vi "Get Project Info.vi"(8 "error in (no error)":errorcluster, 11 "Project Inspector in":refnum<class "Project Inspector.lvclass">) -> (0 "error out":errorcluster, 1 "Path":path, 2 "Name":string, 3 "Project Inspector out":refnum<class "Project Inspector.lvclass">, 4 "Item Paths":path[](array[path]))   [LabVIEW 2017, in "Cobertura.lvlib" / "Project Inspector.lvclass"]
uses:
  Project Inspector.lvclass
  Project Inspector.lvclass/Project Inspector.ctl
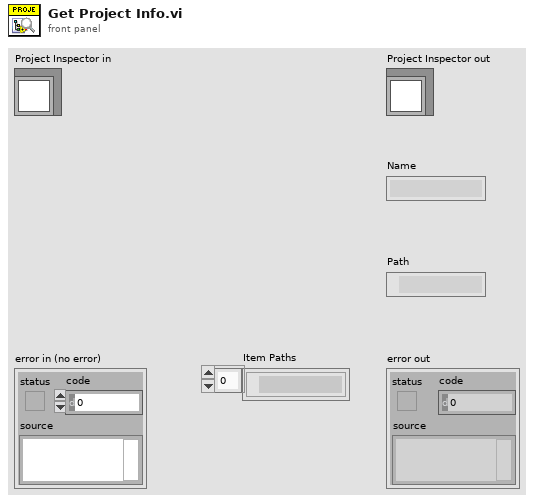
[diagram p1: front panel]
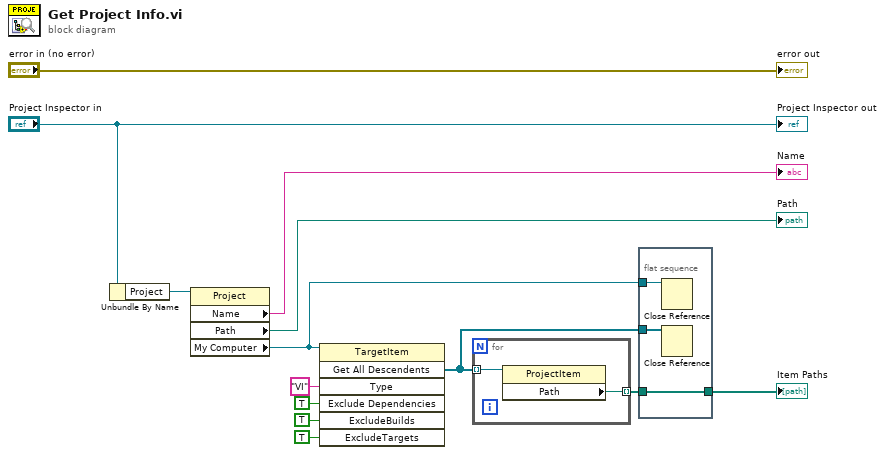
[diagram p0: block diagram]
diagram:
  n1 = Unbundle By Name("Project Inspector in") -> ("Project"=w4:refnum<vi>)
  n2 = property class="Project"(reference=w4) -> ("Name"=→"Name":string, "Path"=→"Path":path, "My Computer"=w6:refnum<vi>)  [unwired: 1 in, 2 out]
  n3 = invoke class="TargetItem" method="Get All Descendents"(reference=w6, "Type"="VI", "Exclude Dependencies"=TRUE ("ExcludeDependencies"), "ExcludeBuilds"=TRUE, "ExcludeTargets"=TRUE) -> ("All Descendents"=w8:refnum<vi>[])  [unwired: 2 in, 6 out]
  n4 = for {
    tunnel: w8 -> [w15] mode=indexing
    tunnel: [w14] -> w7 mode=indexing
    n5 = property class="ProjectItem"(reference=w15) -> ("Path"=w14:path)  [unwired: 1 in, 2 out]
  }
  n6 = flat-sequence {
    tunnel: w8 -> [w18]
    tunnel: [w17] -> w3
    tunnel: w7 -> [w17]
    tunnel: w6 -> [w16]
    frame #0 {
      n7 = Close Reference(reference=w16) -> ()  [unwired: 1 in, 1 out]
      n8 = Close Reference(reference=w18) -> ()  [unwired: 1 in, 1 out]
    }
  }
  "error out" <- "error in (no error)"
  "Project Inspector out" <- "Project Inspector in"
  "Item Paths" <- w3
